vi "read inputs.vi"(11 "inputs":T1[](array[typedef]) format="%.0x") -> (0 "code":i32, 3 "model inputs":T2)   [LabVIEW 2014, in "Scriptable Model Interface Engine.lvlib"]
uses:
  Scriptable Model Interface Engine.lvlib
  Shared/model inputs.ctl
  Shared/Scriptable Model Interface Shared.lvlib
  <vilib>/NI Veristand/Custom Device API/Custom Device API.lvlib
  <vilib>/NI Veristand/Custom Device API/Data Reference.ctl
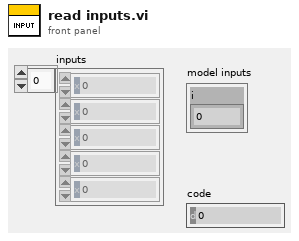
[diagram p1: front panel]
types:
  T1 = typedef "Custom Device API.lvlib/Data Reference.ctl" = i32
  T2 = typedef "Scriptable Model Interface Shared.lvlib/model inputs.ctl" = cluster{"i":dbl}
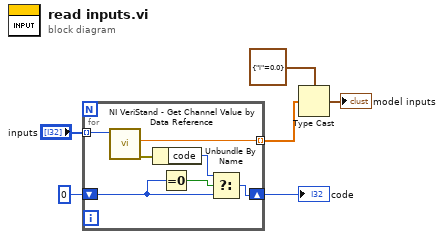
[diagram p0: block diagram]
diagram:
  n1 = for {
    shift-right: [w11] -> w1
    shift-left: 0 ("code") -> [w10]
    tunnel: [w8] -> w3 mode=indexing
    tunnel: "inputs" -> [w7] mode=indexing
    n2 = call <vilib>:"NI VeriStand - Get Channel Value by Data Reference.vi"("Data Reference in"=w7) -> ("error out"=w9:errorcluster, "Value"=w8:dbl)  [unwired: 9 in]
    n3 = Unbundle By Name(w9) -> ("code"=w12:i32)
    n4 = Equal To 0?(x=w10) -> (x = 0?=w13:bool)
    n5 = Select(t=w12, s=w13, f=w10) -> (s? t:f=w11:i32)
  }
  "code" <- w1
  n6 = Type Cast(type=T2 {"i"=0.0} ("model inputs"), x=w3) -> (*(type *) &x=→"model inputs":T2)
